vi "_mzData Convert Array.vi"(3 "Array":dbl[](array[numeric])) -> (0 "String":string, 1 "Length":i32)   [LabVIEW 2012]
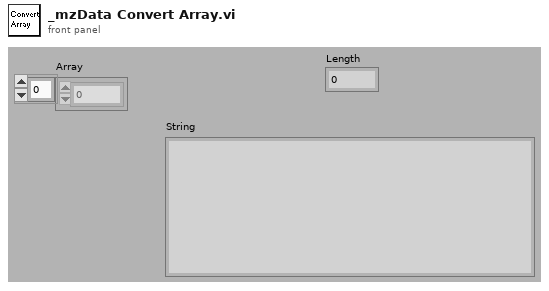
[diagram p1: front panel]
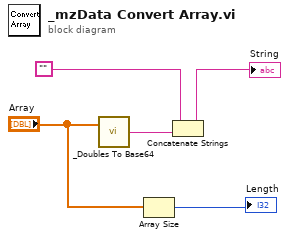
[diagram p0: block diagram]
diagram:
  n1 = call "_Doubles To Base64.vi"("Doubles"="Array") -> ("Base64 String"=w1:string)  [unwired: 1 in]
  n2 = Array Size(array="Array") -> (size(s)=→"Length":i32)
  n3 = Concatenate Strings("", w1) -> (→"String":string)
